vi "TimEtchLoad.vi"(7 "Analyte1":string, 8 "Speed1":dbl, 9 "volume_uL":dbl, 10 "Pump in":refnum<k24>) -> ()   [LabVIEW 2020]
uses:
  D:/PumpAutomation2/DEMPBot2/PumpAdapter.exe
  PumpAdapter.exe
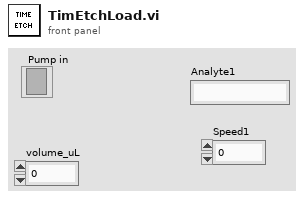
[diagram p1: front panel]
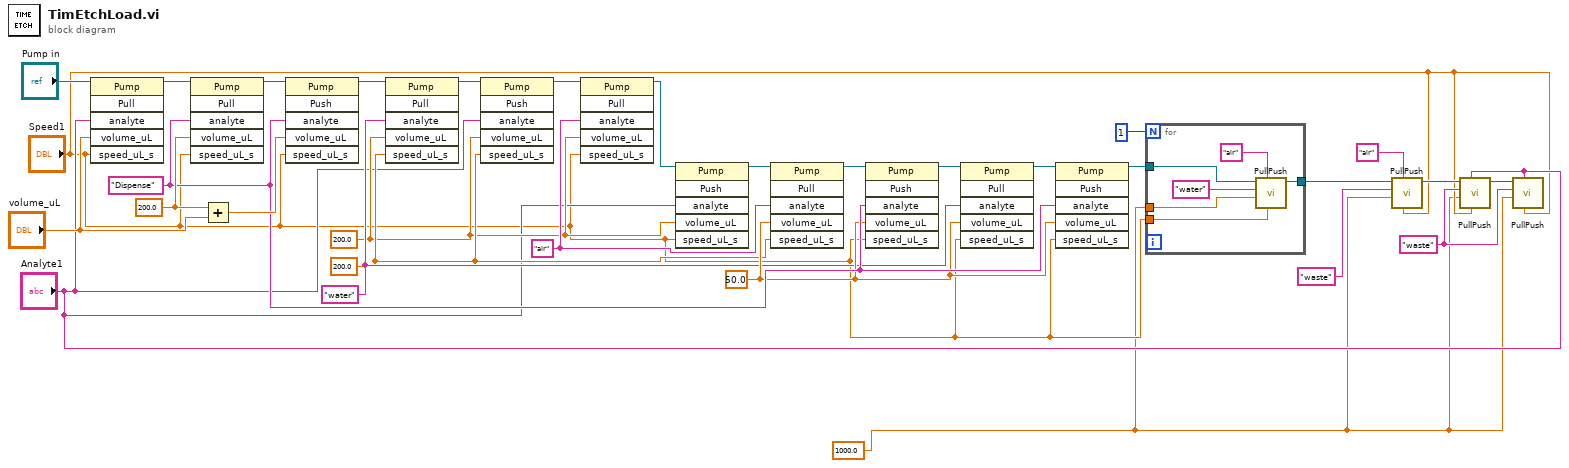
[diagram p0: block diagram]
diagram:
  w1 = 1000.0 ("volume_uL")
  w4 = "waste" ("pullFrom")
  w31 = 200.0 ("volume_uL")
  w27 = 50.0 ("volume_uL")
  w12 = "air" ("analyte")
  w21 = 200.0 ("speed_uL_s")
  w8 = 200.0 ("volume_uL")
  w25 = "water" ("analyte")
  w29 = "Dispense" ("analyte")
  n1 = invoke class="Pump" method="Pull"(reference="Pump in", "analyte"="Analyte1", "volume_uL"="volume_uL", "speed_uL_s"="Speed1") -> (reference out=w14:refnum<k24>)  [unwired: 2 in, 5 out]
  n2 = invoke class="Pump" method="Pull"(reference=w14, "analyte"=w29, "volume_uL"=w31, "speed_uL_s"="Speed1") -> (reference out=w28:refnum<k24>)  [unwired: 2 in, 5 out]
  n3 = Add(x=w31, y="volume_uL") -> (x+y=w30:dbl)
  n4 = invoke class="Pump" method="Push"(reference=w28, "analyte"=w29, "volume_uL"=w30, "speed_uL_s"="Speed1") -> (reference out=w18:refnum<k24>)  [unwired: 2 in, 5 out]
  n5 = invoke class="Pump" method="Pull"(reference=w18, "analyte"=w25, "volume_uL"=w8, "speed_uL_s"=w21) -> (reference out=w20:refnum<k24>)  [unwired: 2 in, 5 out]
  n6 = invoke class="Pump" method="Push"(reference=w20, "analyte"="Analyte1", "volume_uL"=w8, "speed_uL_s"=w21) -> (reference out=w10:refnum<k24>)  [unwired: 2 in, 5 out]
  n7 = invoke class="Pump" method="Pull"(reference=w10, "analyte"=w12, "volume_uL"=w8, "speed_uL_s"="Speed1") -> (reference out=w11:refnum<k24>)  [unwired: 2 in, 5 out]
  n8 = invoke class="Pump" method="Push"(reference=w11, "analyte"="Analyte1", "volume_uL"=w8, "speed_uL_s"="Speed1") -> (reference out=w9:refnum<k24>)  [unwired: 2 in, 5 out]
  n9 = invoke class="Pump" method="Pull"(reference=w9, "analyte"=w12, "volume_uL"=w27, "speed_uL_s"=w21) -> (reference out=w22:refnum<k24>)  [unwired: 2 in, 5 out]
  n10 = invoke class="Pump" method="Push"(reference=w22, "analyte"=w29, "volume_uL"=w27, "speed_uL_s"="Speed1") -> (reference out=w23:refnum<k24>)  [unwired: 2 in, 5 out]
  n11 = invoke class="Pump" method="Pull"(reference=w23, "analyte"=w25, "volume_uL"=w27, "speed_uL_s"="Speed1") -> (reference out=w24:refnum<k24>)  [unwired: 2 in, 5 out]
  n12 = invoke class="Pump" method="Push"(reference=w24, "analyte"=w29, "volume_uL"=w27, "speed_uL_s"="Speed1") -> (reference out=w26:refnum<k24>)  [unwired: 2 in, 5 out]
  n13 = for {
    N: 1 -> [_]
    tunnel: w26 -> [w37]
    tunnel: w1 -> [w35]
    tunnel: "Speed1" -> [w34]
    tunnel: [w32] -> w19
    n14 = call "PullPush.vi"("speed_uL_s"=w34, "pushTo"="air", "volume_uL"=w35, "pullFrom"="water", ".NET Refnum in"=w37) -> (".NET Refnum out"=w32:refnum<k24>)  [unwired: 6 in]
  }
  n15 = call "PullPush.vi"("speed_uL_s"="Speed1", "pushTo"="air", "volume_uL"=w1, "pullFrom"="waste", ".NET Refnum in"=w19) -> (".NET Refnum out"=w6:refnum<k24>)  [unwired: 6 in]
  n16 = call "PullPush.vi"("speed_uL_s"="Speed1", "pushTo"="Analyte1", "volume_uL"=w1, "pullFrom"=w4, ".NET Refnum in"=w6) -> (".NET Refnum out"=w5:refnum<k24>)  [unwired: 6 in]
  n17 = call "PullPush.vi"("speed_uL_s"="Speed1", "pushTo"="Analyte1", "volume_uL"=w1, "pullFrom"=w4, ".NET Refnum in"=w5) -> ()  [unwired: 6 in, 1 out]
